vi "testing_readSingleCount.vi"() -> ()   [LabVIEW 2015, in "Tausand AB1000.lvlib"]
uses:
  <instrlib>/Tausand AB1000/Tausand AB1000.lvlib
  <instrlib>/Tausand AB1000/Public/Controls/deviceTypeRing.ctl
  <instrlib>/Tausand AB1000/Public/Controls/channelRing.ctl
  <vilib>/Analysis/baseanly.llb/Mean (DBL).vi
  <vilib>/Analysis/NI_AALBase.lvlib
panel:
  in  "channel (A=1)":T1=1 items=["none", "A", "B", "C", "D", "E", "F", "G", "H"]
  out "value":u32
  out "label":string
  out "min reading timer (s)":dbl format="%0.4f"
  out "max reading timer (s)":dbl format="%0.4f"
  out "reading timer mean (s)":dbl format="%0.4f"
  out "reading timer histogram":T2(graph)
  in  "stop":bool
  out "last reading timer (s)":dbl format="%0.4f"
  out "error out":errorcluster
  in  "VISA resource name":refnum<visa-resource-name>
  in  "error in (no error)":errorcluster
  out "checksum ok?":bool
  out "read time":timestamp
  in  "read timeout (500 ms)":u32=500
  in  "device type":T3 items=["any"=0, "AB1002"=1002, "AB1004"=1004, "AB1502"=1502, "AB1504"=1504, "AB1902"=1902, "AB1904"=1904, "AB2002"=2002, "AB2004"=2004, "AB2502"=2502, "AB2504"=2504, "AB2902"=2902, "AB2904"=2904]
  # "TEST of: 'Read single counter.vi'"
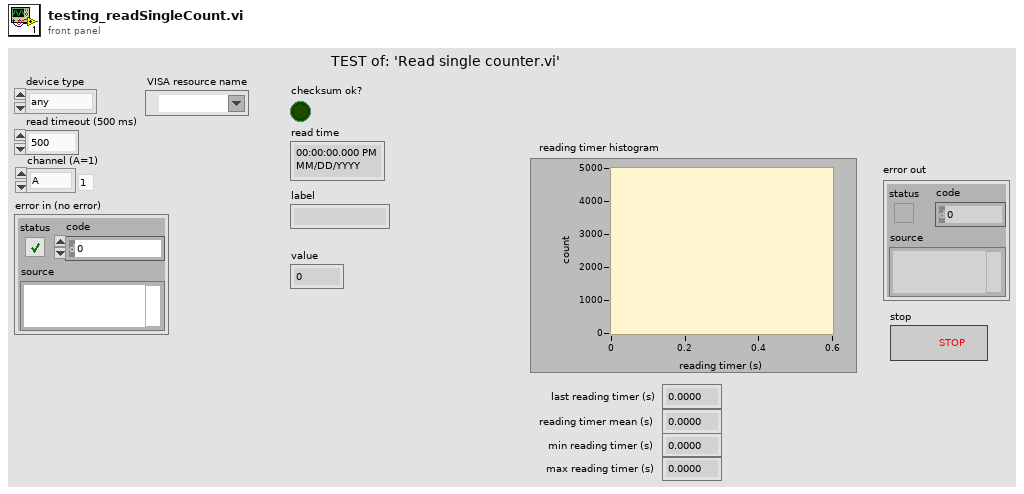
[diagram p1: front panel]
types:
  T1 = typedef "Tausand AB1000.lvlib/channelRing.ctl" = u8
  T2 = cluster{"X Values":dbl[], "Histogram: h(x)":i32[]}
  T3 = typedef "Tausand AB1000.lvlib/deviceTypeRing.ctl" = u16
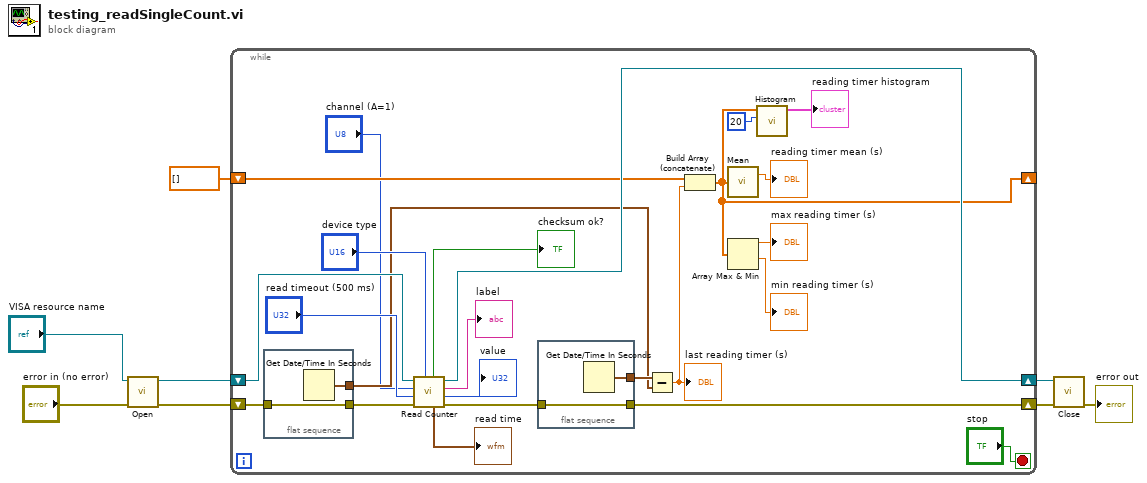
[diagram p0: block diagram]
diagram:
  n1 = call <instrlib>:"Open.vi"("error in (no error)"="error in (no error)", "VISA resource name"="VISA resource name") -> ("error out"=w3:errorcluster, "VISA resource name out"=w8:refnum<visa-resource-name>)  [unwired: 8 in]
  n2 = while {
    shift-right: [w31] -> w7
    shift-left: w8 -> [w32]
    shift-right: [w23] -> w2
    shift-left: w3 -> [w25]
    shift-right: [w14] -> _
    shift-left: dbl[] [] -> [w18]
    stop <- "stop" stop-if-true
    n3 = flat-sequence {
      tunnel: [w36] -> w26
      tunnel: w25 -> [w36]
      tunnel: [w35] -> w21
      frame #0 {
        n4 = Get Date/Time In Seconds() -> (seconds since 1Jan1904=w35:timestamp)
      }
    }
    n5 = call <instrlib>:"Read Counter.vi"("device type"="device type", "error in (no error)"=w26, "read timeout (500 ms)"="read timeout (500 ms)", "channel (A=1)"="channel (A=1)", "VISA Refnum in"=w32) -> ("error out"=w24:errorcluster, "value"=→"value":u32, "label"=→"label":string, "VISA Refnum out"=w31:refnum<visa-resource-name>, "read time"=→"read time":timestamp, "checksum ok?"=→"checksum ok?":bool)  [unwired: 1 in]
    n6 = flat-sequence {
      tunnel: [w34] -> w23
      tunnel: w24 -> [w34]
      tunnel: [w33] -> w22
      frame #0 {
        n7 = Get Date/Time In Seconds() -> (seconds since 1Jan1904=w33:timestamp)
      }
    }
    n8 = Subtract(x=w22, y=w21) -> (x-y=w19:dbl)
    "last reading timer (s)" <- w19
    n9 = Build Array (concatenate)(w18, w19) -> (w14:dbl[])
    n10 = call-poly <vilib>:"Mean.vi"("X"=w14) -> ("mean"=→"reading timer mean (s)":dbl)  [unwired: 1 out]
    n11 = Array Max & Min(array=w14) -> (max value=→"max reading timer (s)":dbl, min value=→"min reading timer (s)":dbl)  [unwired: 2 out]
    n12 = call <vilib>:"Histogram.vi"("intervals"=20, "X"=w14) -> ("Histogram Graph"=→"reading timer histogram":T2)  [unwired: 6 in, 3 out]
  }
  n13 = call <instrlib>:"Close.vi"("error in (no error)"=w2, "VISA resource name"=w7) -> ("error out"=→"error out":errorcluster)  [unwired: 9 in]
